vi "Velocity Drive.vi"(7 "High Gear?":bool, 8 "error in (no error)":errorcluster, 9 "Right Speed":dbl, 10 "Left Speed":dbl, 11 "Falcon500 in":refnum<class "Falcon500.lvclass">) -> (0 "error out":errorcluster, 3 "Falcon500 out":refnum<class "Falcon500.lvclass">)   [LabVIEW 2019, in "Drive.lvlib" / "Falcon500.lvclass"]
doc: "switches into velocity drive"
uses:
  Falcon500.lvclass
  C:/Users/Public/Documents/2020InfinteRecharge/src robot/Classes/Drive/Tank Drive/Tank Drive.lvclass
  <vilib>/Rock Robotics/WPI/ThirdParty/Phoenix-LabVIEW/Motor Controller/Controls/CTRE_Phoenix_MotorControl_ControlMode.ctl
  <vilib>/Rock Robotics/Network Tables/NT Read Boolean.vi
panel:
  in  "High Gear Max Velocity":dbl=30000.0
  in  "Low Gear Max Velocity":dbl=15000.0
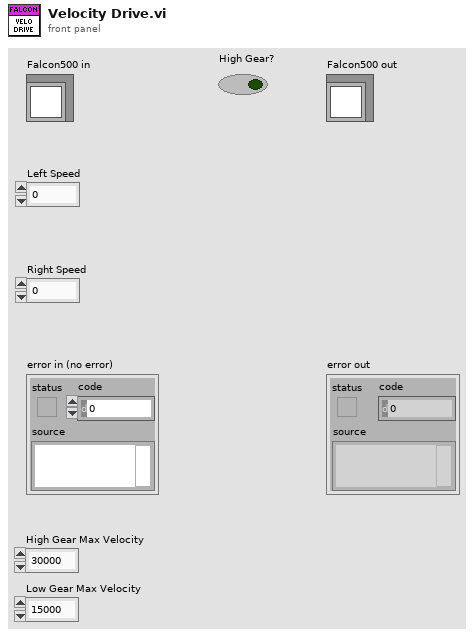
[diagram p1: front panel]
types:
  T1 = typedef "CTRE_Phoenix_MotorControl_ControlMode.ctl" = u16
  T2 = typedef "Drive.lvlib/Tank Drive.lvclass/Motor Controller Names.ctl" = cluster{"Left Lead":string, "Right Lead":string, "Left Followers":string[], "Right Followers":string[]}
  T3 = typedef "WPI_MotorControlDeviceRef.ctl" = cluster{"DeviceStatus":errorcluster, "Type":T4, "PWM":cluster{"PWM Channel":T5, "DeadBand":T6}, "CAN":cluster{"Device Number":u8, "SetOutput VI Ref":variant, "GetOutput VI Ref":variant, "Enable VI Ref":variant, "Disable VI Ref":variant, "Data":variant}, "Invert":bool, "DIO PWM":cluster{"PWM \"Enable\" Channel":T5, "DIOChannel":T7, "PWM Rate":dbl}}
  T4 = typedef "WPI_MotorControlType.ctl" = enum16{"PWM", "CAN", "DIO PWM"}
  T5 = typedef "FPGA_DIOPWMChannel.ctl" = enum8{"PWM 0", "PWM 1", "PWM 2", "PWM 3", "PWM 4", "PWM 5", "PWM 6", "PWM 7", "PWM 8", "PWM 9", "PWM MXP 0", "PWM MXP 1", "PWM MXP 2", "PWM MXP 3", "PWM MXP 4", "PWM MXP 5", "PWM MXP 6", "PWM MXP 7", "PWM MXP 8", "PWM MXP 9", "Invalid"}
  T6 = typedef "WPI_PWMDeadband.ctl" = cluster{"Name":string, "maxPositivePwm":i32, "minPositivePwm":i32, "centerPwm":i32, "maxNegativePwm":i32, "minNegativePwm":i32, "angularRange":u16}
  T7 = typedef "FPGA_DIOChannel.ctl" = enum8{"DIO 0", "DIO 1", "DIO 2", "DIO 3", "DIO 4", "DIO 5", "DIO 6", "DIO 7", "DIO 8", "DIO 9", "DIO MXP 0", "DIO MXP 1", "DIO MXP 2", "DIO MXP 3", "DIO MXP 4", "DIO MXP 5", "DIO MXP 6", "DIO MXP 7", "DIO MXP 8", "DIO MXP 9", "DIO MXP 10", "DIO MXP 11", "DIO MXP 12", "DIO MXP 13", "DIO MXP 14", "DIO MXP 15", "SPI Port CS1", "SPI Port CS2", "SPI Port CS3", "SPI Port MISO", "SPI Port MOSI", "Invalid"}
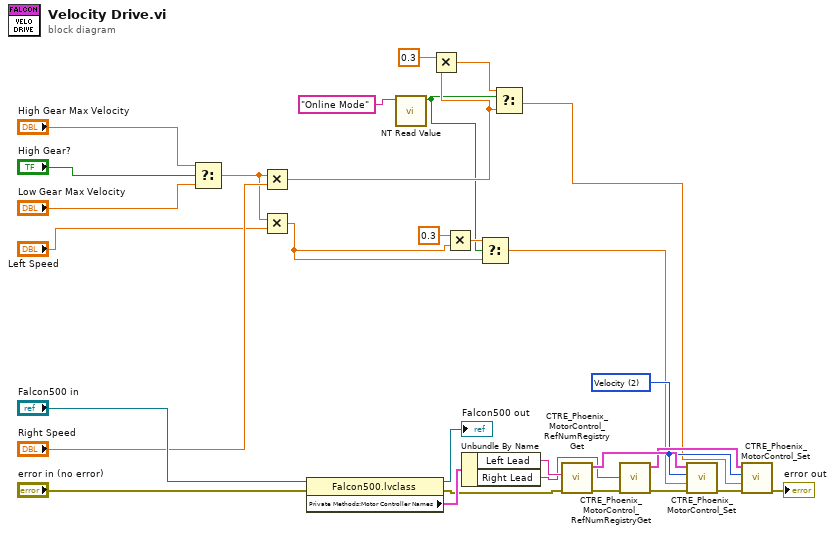
[diagram p0: block diagram]
diagram:
  w20 = T1 2 items=["PercentOutput"=0, "Position"=1, "Velocity"=2, "Current"=3, "Follower"=5, "MotionProfile"=6, "MotionMagic"=7, "MotionProfileArc"=10, "Disabled"=15] ("Control Mode")
  n1 = Select(t="High Gear Max Velocity", s="High Gear?", f="Low Gear Max Velocity") -> (s? t:f=w12:dbl)
  n2 = Multiply(x=w12, y="Right Speed") -> (x*y=w6:dbl)
  n3 = Multiply(x=w12, y="Left Speed") -> (x*y=w3:dbl)
  n4 = property class="Falcon500.lvclass"(reference="Falcon500 in", error in="error in (no error)") -> (reference out=→"Falcon500 out":refnum<class "Falcon500.lvclass">, error out=w17:errorcluster, "Private Methods:Motor Controller Names"=w30:T2)
  n5 = call-poly <vilib>:"NT Read Value.vi"("Name"="Online Mode") -> ("Boolean"=w1:bool)  [unwired: 9 in, 1 out]
  n6 = Multiply(x=0.3, y=w6) -> (x*y=w8:dbl)
  n7 = Multiply(x=0.3, y=w3) -> (x*y=w2:dbl)
  n8 = Unbundle By Name(w30) -> ("Left Lead"=w27:string, "Right Lead"=w18:string)
  n9 = Select(t=w2, s=w1, f=w3) -> (s? t:f=w5:dbl)
  n10 = Select(t=w8, s=w1, f=w6) -> (s? t:f=w9:dbl)
  n11 = call <vilib>:"CTRE_Phoenix_MotorControl_RefNumRegistryGet.vi"("error in (no error)"=w17, "refnum name"=w27) -> ("error out"=w26:errorcluster, "PhoenixMotorControlDevRef"=w24:T3)  [unwired: 8 in]
  n12 = call <vilib>:"CTRE_Phoenix_MotorControl_RefNumRegistryGet.vi"("error in (no error)"=w26, "refnum name"=w18) -> ("error out"=w22:errorcluster, "PhoenixMotorControlDevRef"=w23:T3)  [unwired: 8 in]
  n13 = call <vilib>:"CTRE_Phoenix_MotorControl_Set.vi"("error in (no error)"=w22, "Output"=w5, "Control Mode"=w20, "PhoenixMotorControlDevRef"=w24) -> ("error out"=w25:errorcluster)  [unwired: 6 in, 1 out]
  n14 = call <vilib>:"CTRE_Phoenix_MotorControl_Set.vi"("error in (no error)"=w25, "Output"=w9, "Control Mode"=w20, "PhoenixMotorControlDevRef"=w23) -> ("error out"=→"error out":errorcluster)  [unwired: 6 in, 1 out]
